vi "Adaptive Filter ECG.vi"(4 "Beta":fxp<+/-,32,-16> format="%.44g", 5 "Beta IBP":fxp<+/-,32,-16> format="%.44g", 6 "Filter Length":i32, 8 "Data in":T5, 11 "Memory Blocks In":T3) -> (0 "Data":T2 {"BetaProduct" format="%.33g"; "WeightSum" format="%.20g"}, 1 "IBP Out":cluster{"IBP0":i16, "IBP1":i16}, 2 "Filtered Leads":T1, 3 "Raw Leads":T1)   [LabVIEW 2017]
uses:
  Memory Block Channels.ctl
  MemoryBlocks.ctl
  ECG Leads.ctl
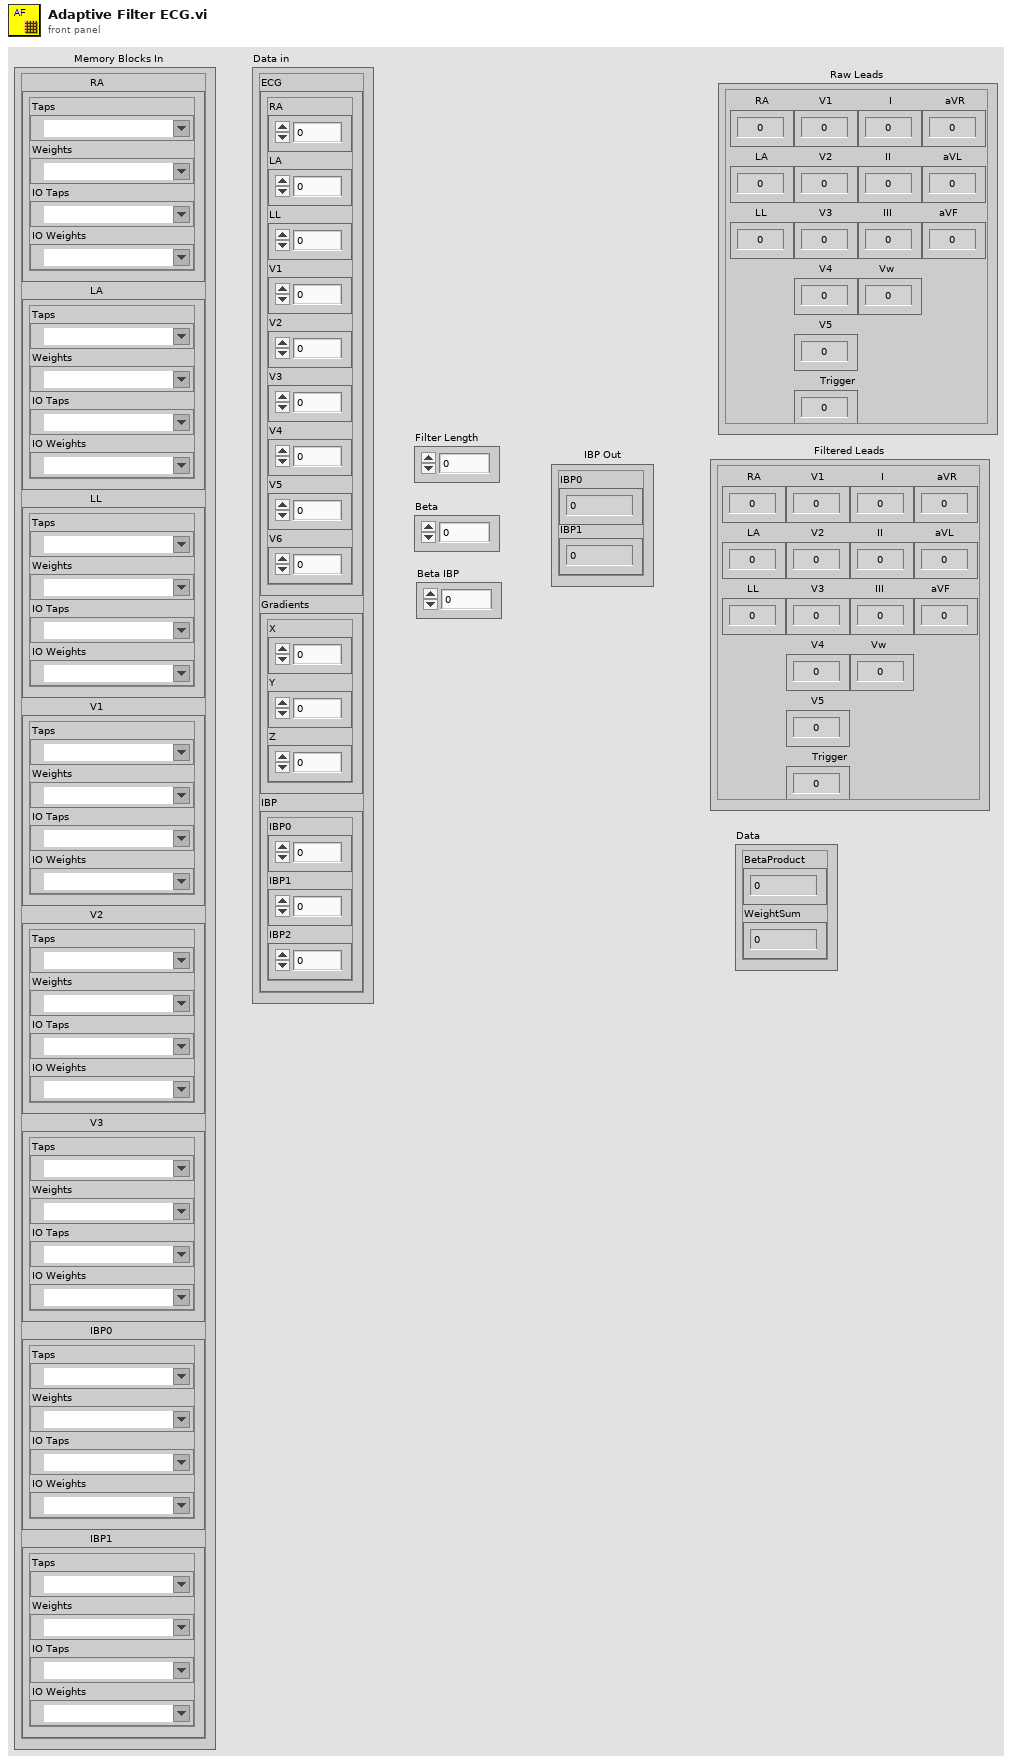
[diagram p1: front panel]
types:
  T1 = typedef "ECG Leads.ctl" = cluster{"RA":i16, "LA":i16, "LL":i16, "V1":i16, "V2":i16, "V3":i16, "V4":i16, "V5":i16, "Trigger":i16, "I":i16, "II":i16, "III":i16, "aVR":i16, "aVL":i16, "aVF":i16, "Vw":i16}
  T2 = cluster{"BetaProduct":fxp<+/-,32,-1>, "WeightSum":fxp<+/-,33,19>}
  T3 = typedef "Memory Block Channels.ctl" = cluster{"RA":T4, "LA":T4, "LL":T4, "V1":T4, "V2":T4, "V3":T4, "IBP0":T4, "IBP1":T4}
  T4 = typedef "MemoryBlocks.ctl" = cluster{"Taps":refnum<k21>, "Weights":refnum<k21>, "IO Weights":refnum<k21>, "IO Taps":refnum<k21>}
  T5 = cluster{"ECG":cluster{"RA":fxp<+/-,16,16>, "LA":fxp<+/-,16,16>, "LL":fxp<+/-,16,16>, "V1":fxp<+/-,16,16>, "V2":fxp<+/-,16,16>, "V3":fxp<+/-,16,16>, "V4":fxp<+/-,16,16>, "V5":fxp<+/-,16,16>, "V6":fxp<+/-,16,16>}, "Gradients":cluster{"X":fxp<+/-,16,16>, "Y":fxp<+/-,16,16>, "Z":fxp<+/-,16,16>}, "IBP":cluster{"IBP0":fxp<+/-,16,16>, "IBP1":fxp<+/-,16,16>, "IBP2":fxp<+/-,16,16>}}
  T6 = cluster{"RA":fxp<+/-,16,16>, "LA":fxp<+/-,16,16>, "LL":fxp<+/-,16,16>, "V1":fxp<+/-,16,16>, "V2":fxp<+/-,16,16>, "V3":fxp<+/-,16,16>, "V4":fxp<+/-,16,16>, "V5":fxp<+/-,16,16>, "V6":fxp<+/-,16,16>}
  T7 = cluster{"X":fxp<+/-,16,16>, "Y":fxp<+/-,16,16>, "Z":fxp<+/-,16,16>}
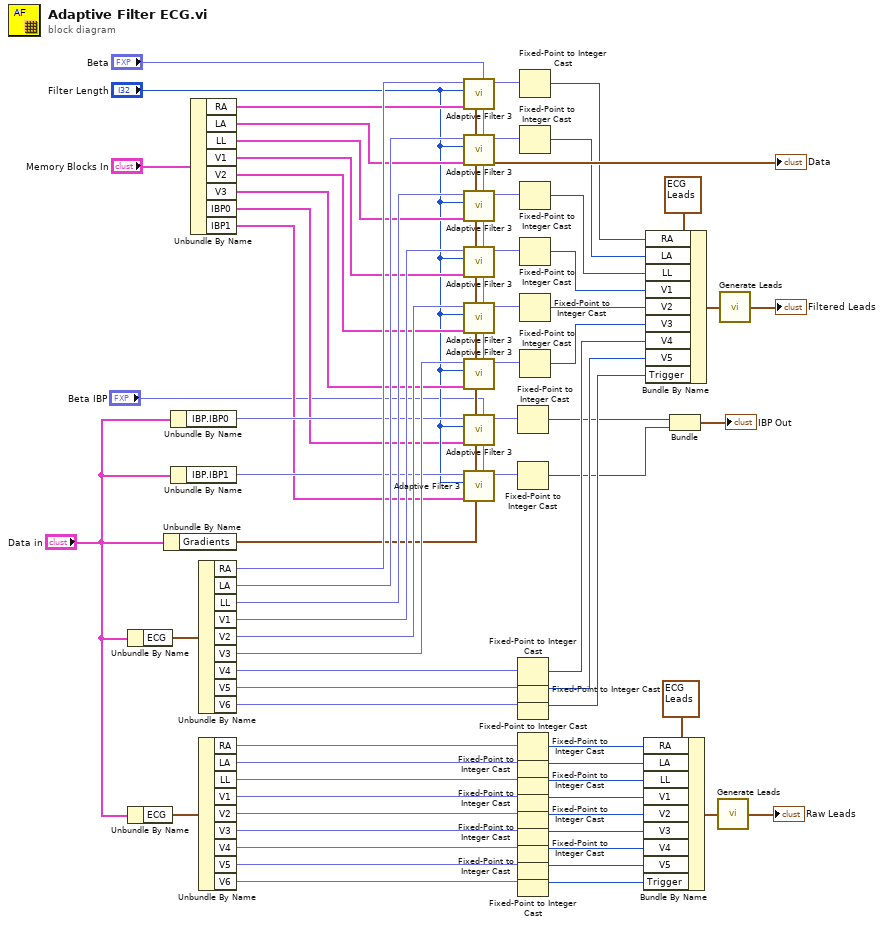
[diagram p0: block diagram]
diagram:
  n1 = Unbundle By Name("Data in") -> ("ECG"=w48:T6)
  n2 = Unbundle By Name("Data in") -> ("ECG"=w55:T6)
  n3 = Unbundle By Name("Data in") -> ("Gradients"=w13:T7)
  n4 = Unbundle By Name("Data in") -> ("IBP.IBP0"=w14:fxp<+/-,16,16>)
  n5 = Unbundle By Name("Data in") -> ("IBP.IBP1"=w11:fxp<+/-,16,16>)
  n6 = Unbundle By Name("Memory Blocks In") -> ("RA"=w42:T4, "LA"=w43:T4, "LL"=w44:T4, "V1"=w45:T4, "V2"=w46:T4, "V3"=w47:T4, "IBP0"=w8:T4, "IBP1"=w7:T4)
  n7 = Unbundle By Name(w48) -> ("RA"=w49:fxp<+/-,16,16>, "LA"=w50:fxp<+/-,16,16>, "LL"=w51:fxp<+/-,16,16>, "V1"=w52:fxp<+/-,16,16>, "V2"=w53:fxp<+/-,16,16>, "V3"=w54:fxp<+/-,16,16>, "V4"=w18:fxp<+/-,16,16>, "V5"=w19:fxp<+/-,16,16>, "V6"=w20:fxp<+/-,16,16>)
  n8 = Unbundle By Name(w55) -> ("RA"=w56:fxp<+/-,16,16>, "LA"=w57:fxp<+/-,16,16>, "LL"=w58:fxp<+/-,16,16>, "V1"=w59:fxp<+/-,16,16>, "V2"=w60:fxp<+/-,16,16>, "V3"=w61:fxp<+/-,16,16>, "V4"=w62:fxp<+/-,16,16>, "V5"=w63:fxp<+/-,16,16>, "V6"=w64:fxp<+/-,16,16>)
  n9 = call "Adaptive Filter 3.vi"("Beta"="Beta", "Noise"=w13, "Memory"=w42, "Filter Size"="Filter Length", "Input"=w49) -> ("Error Out"=w24:fxp<+/-,16,16>)  [unwired: 5 in, 1 out]
  n10 = call "Adaptive Filter 3.vi"("Beta"="Beta", "Noise"=w13, "Memory"=w43, "Filter Size"="Filter Length", "Input"=w50) -> ("Data"=→"Data":T2, "Error Out"=w25:fxp<+/-,16,16>)  [unwired: 5 in]
  n11 = call "Adaptive Filter 3.vi"("Beta"="Beta", "Noise"=w13, "Memory"=w44, "Filter Size"="Filter Length", "Input"=w51) -> ("Error Out"=w26:fxp<+/-,16,16>)  [unwired: 5 in, 1 out]
  n12 = call "Adaptive Filter 3.vi"("Beta"="Beta", "Noise"=w13, "Memory"=w45, "Filter Size"="Filter Length", "Input"=w52) -> ("Error Out"=w27:fxp<+/-,16,16>)  [unwired: 5 in, 1 out]
  n13 = call "Adaptive Filter 3.vi"("Beta"="Beta", "Noise"=w13, "Memory"=w46, "Filter Size"="Filter Length", "Input"=w53) -> ("Error Out"=w28:fxp<+/-,16,16>)  [unwired: 5 in, 1 out]
  n14 = call "Adaptive Filter 3.vi"("Beta"="Beta", "Noise"=w13, "Memory"=w47, "Filter Size"="Filter Length", "Input"=w54) -> ("Error Out"=w29:fxp<+/-,16,16>)  [unwired: 5 in, 1 out]
  n15 = call "Adaptive Filter 3.vi"("Beta"="Beta IBP", "Noise"=w13, "Memory"=w8, "Filter Size"="Filter Length", "Input"=w14) -> ("Error Out"=w6:fxp<+/-,16,16>)  [unwired: 5 in, 1 out]
  n16 = call "Adaptive Filter 3.vi"("Beta"="Beta IBP", "Noise"=w13, "Memory"=w7, "Filter Size"="Filter Length", "Input"=w11) -> ("Error Out"=w5:fxp<+/-,16,16>)  [unwired: 5 in, 1 out]
  n17 = Fixed-Point to Integer Cast(1:w6) -> (0:w4:i16)
  n18 = Fixed-Point to Integer Cast(1:w5) -> (0:w3:i16)
  n19 = Fixed-Point to Integer Cast(1:w18) -> (0:w17:i16)
  n20 = Fixed-Point to Integer Cast(1:w19) -> (0:w16:i16)
  n21 = Fixed-Point to Integer Cast(1:w20) -> (0:w15:i16)
  n22 = Fixed-Point to Integer Cast(1:w56) -> (0:w65:i16)
  n23 = Fixed-Point to Integer Cast(1:w57) -> (0:w66:i16)
  n24 = Fixed-Point to Integer Cast(1:w58) -> (0:w67:i16)
  n25 = Fixed-Point to Integer Cast(1:w59) -> (0:w68:i16)
  n26 = Fixed-Point to Integer Cast(1:w60) -> (0:w69:i16)
  n27 = Fixed-Point to Integer Cast(1:w61) -> (0:w70:i16)
  n28 = Fixed-Point to Integer Cast(1:w62) -> (0:w21:i16)
  n29 = Fixed-Point to Integer Cast(1:w63) -> (0:w22:i16)
  n30 = Fixed-Point to Integer Cast(1:w64) -> (0:w23:i16)
  n31 = Fixed-Point to Integer Cast(1:w24) -> (0:w38:i16)
  n32 = Fixed-Point to Integer Cast(1:w25) -> (0:w37:i16)
  n33 = Fixed-Point to Integer Cast(1:w26) -> (0:w36:i16)
  n34 = Fixed-Point to Integer Cast(1:w27) -> (0:w35:i16)
  n35 = Fixed-Point to Integer Cast(1:w28) -> (0:w34:i16)
  n36 = Fixed-Point to Integer Cast(1:w29) -> (0:w39:i16)
  n37 = Bundle By Name(cluster=T1 {"RA"=0, "LA"=0, "LL"=0, "V1"=0, "V2"=0, "V3"=0, "V4"=0, "V5"=0, "Trigger"=0, "I"=0, "II"=0, "III"=0, "aVR"=0, "aVL"=0, "aVF"=0, "Vw"=0} ("Leads"), "RA"=w65, "LA"=w66, "LL"=w67, "V1"=w68, "V2"=w69, "V3"=w70, "V4"=w21, "V5"=w22, "Trigger"=w23) -> (w32:T1)
  n38 = Bundle By Name(cluster=T1 {"RA"=0, "LA"=0, "LL"=0, "V1"=0, "V2"=0, "V3"=0, "V4"=0, "V5"=0, "Trigger"=0, "I"=0, "II"=0, "III"=0, "aVR"=0, "aVL"=0, "aVF"=0, "Vw"=0} ("Leads"), "RA"=w38, "LA"=w37, "LL"=w36, "V1"=w35, "V2"=w34, "V3"=w39, "V4"=w17, "V5"=w16, "Trigger"=w15) -> (w30:T1)
  n39 = Bundle(w4, w3) -> (→"IBP Out":cluster{i16, i16})  [unwired: 1 in]
  n40 = call "Generate Leads.vi"("Leads In"=w32) -> ("Leads Out"=→"Raw Leads":T1)
  n41 = call "Generate Leads.vi"("Leads In"=w30) -> ("Leads Out"=→"Filtered Leads":T1)
